vi "run_weather.vi"() -> ()   [LabVIEW 2011]
uses:
  <vilib>/xml/Load XML File.vi
  <vilib>/xml/Close Reference(Node).vi
  <vilib>/xml/NI_XML.lvlib
panel:
  out "Error Msg":string
  out "Updating Weather":bool
  out "?":picture
  out "Hourly Forecast":string[][](array[string])
  in  "Update Interval (hour)":dbl=1.0
  out "Current Weather":string[][](array[string])
  out "Observation Time (RFC 822)":string
  out "Elevation":string
  out "Longitude":string
  out "Latitude":string
  out "Country (ISO 3166)":string
  out "Location":string
  in  "City":string="stockholm"
  in  "Country":string="sweden"
  out "URL":string
  out "Key ID":string="3b63fd7c50251341"
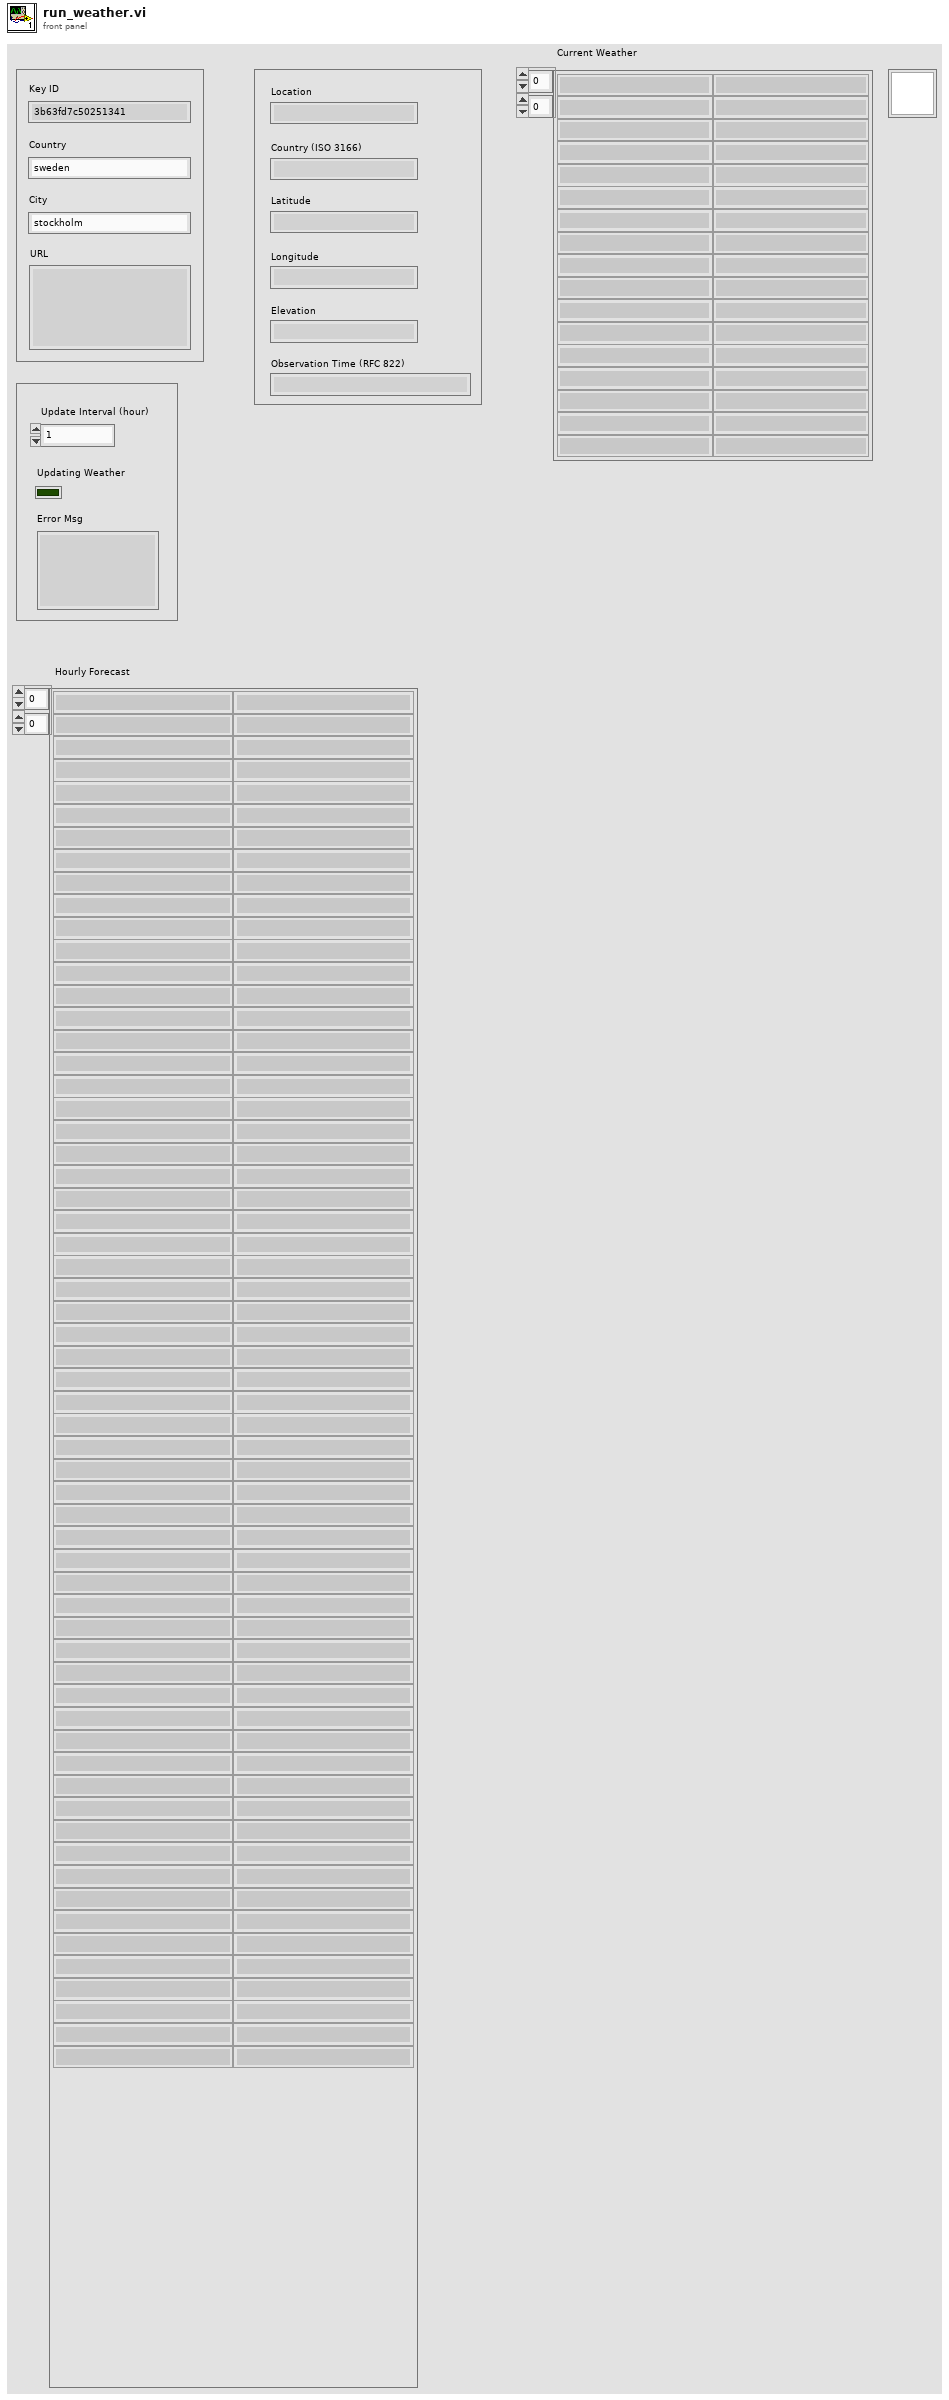
[diagram p1: front panel]
types:
  T1 = enum16{"open", "open or create", "create or replace", "create", "open (read only)"}
  T2 = typedef "imagedata.ctl" = cluster{"image type":i32, "image depth":i32, "image":u8[], "mask":u8[], "colors":u32[], "Rectangle":cluster{"left":i16, "top":i16, "right":i16, "bottom":i16}}
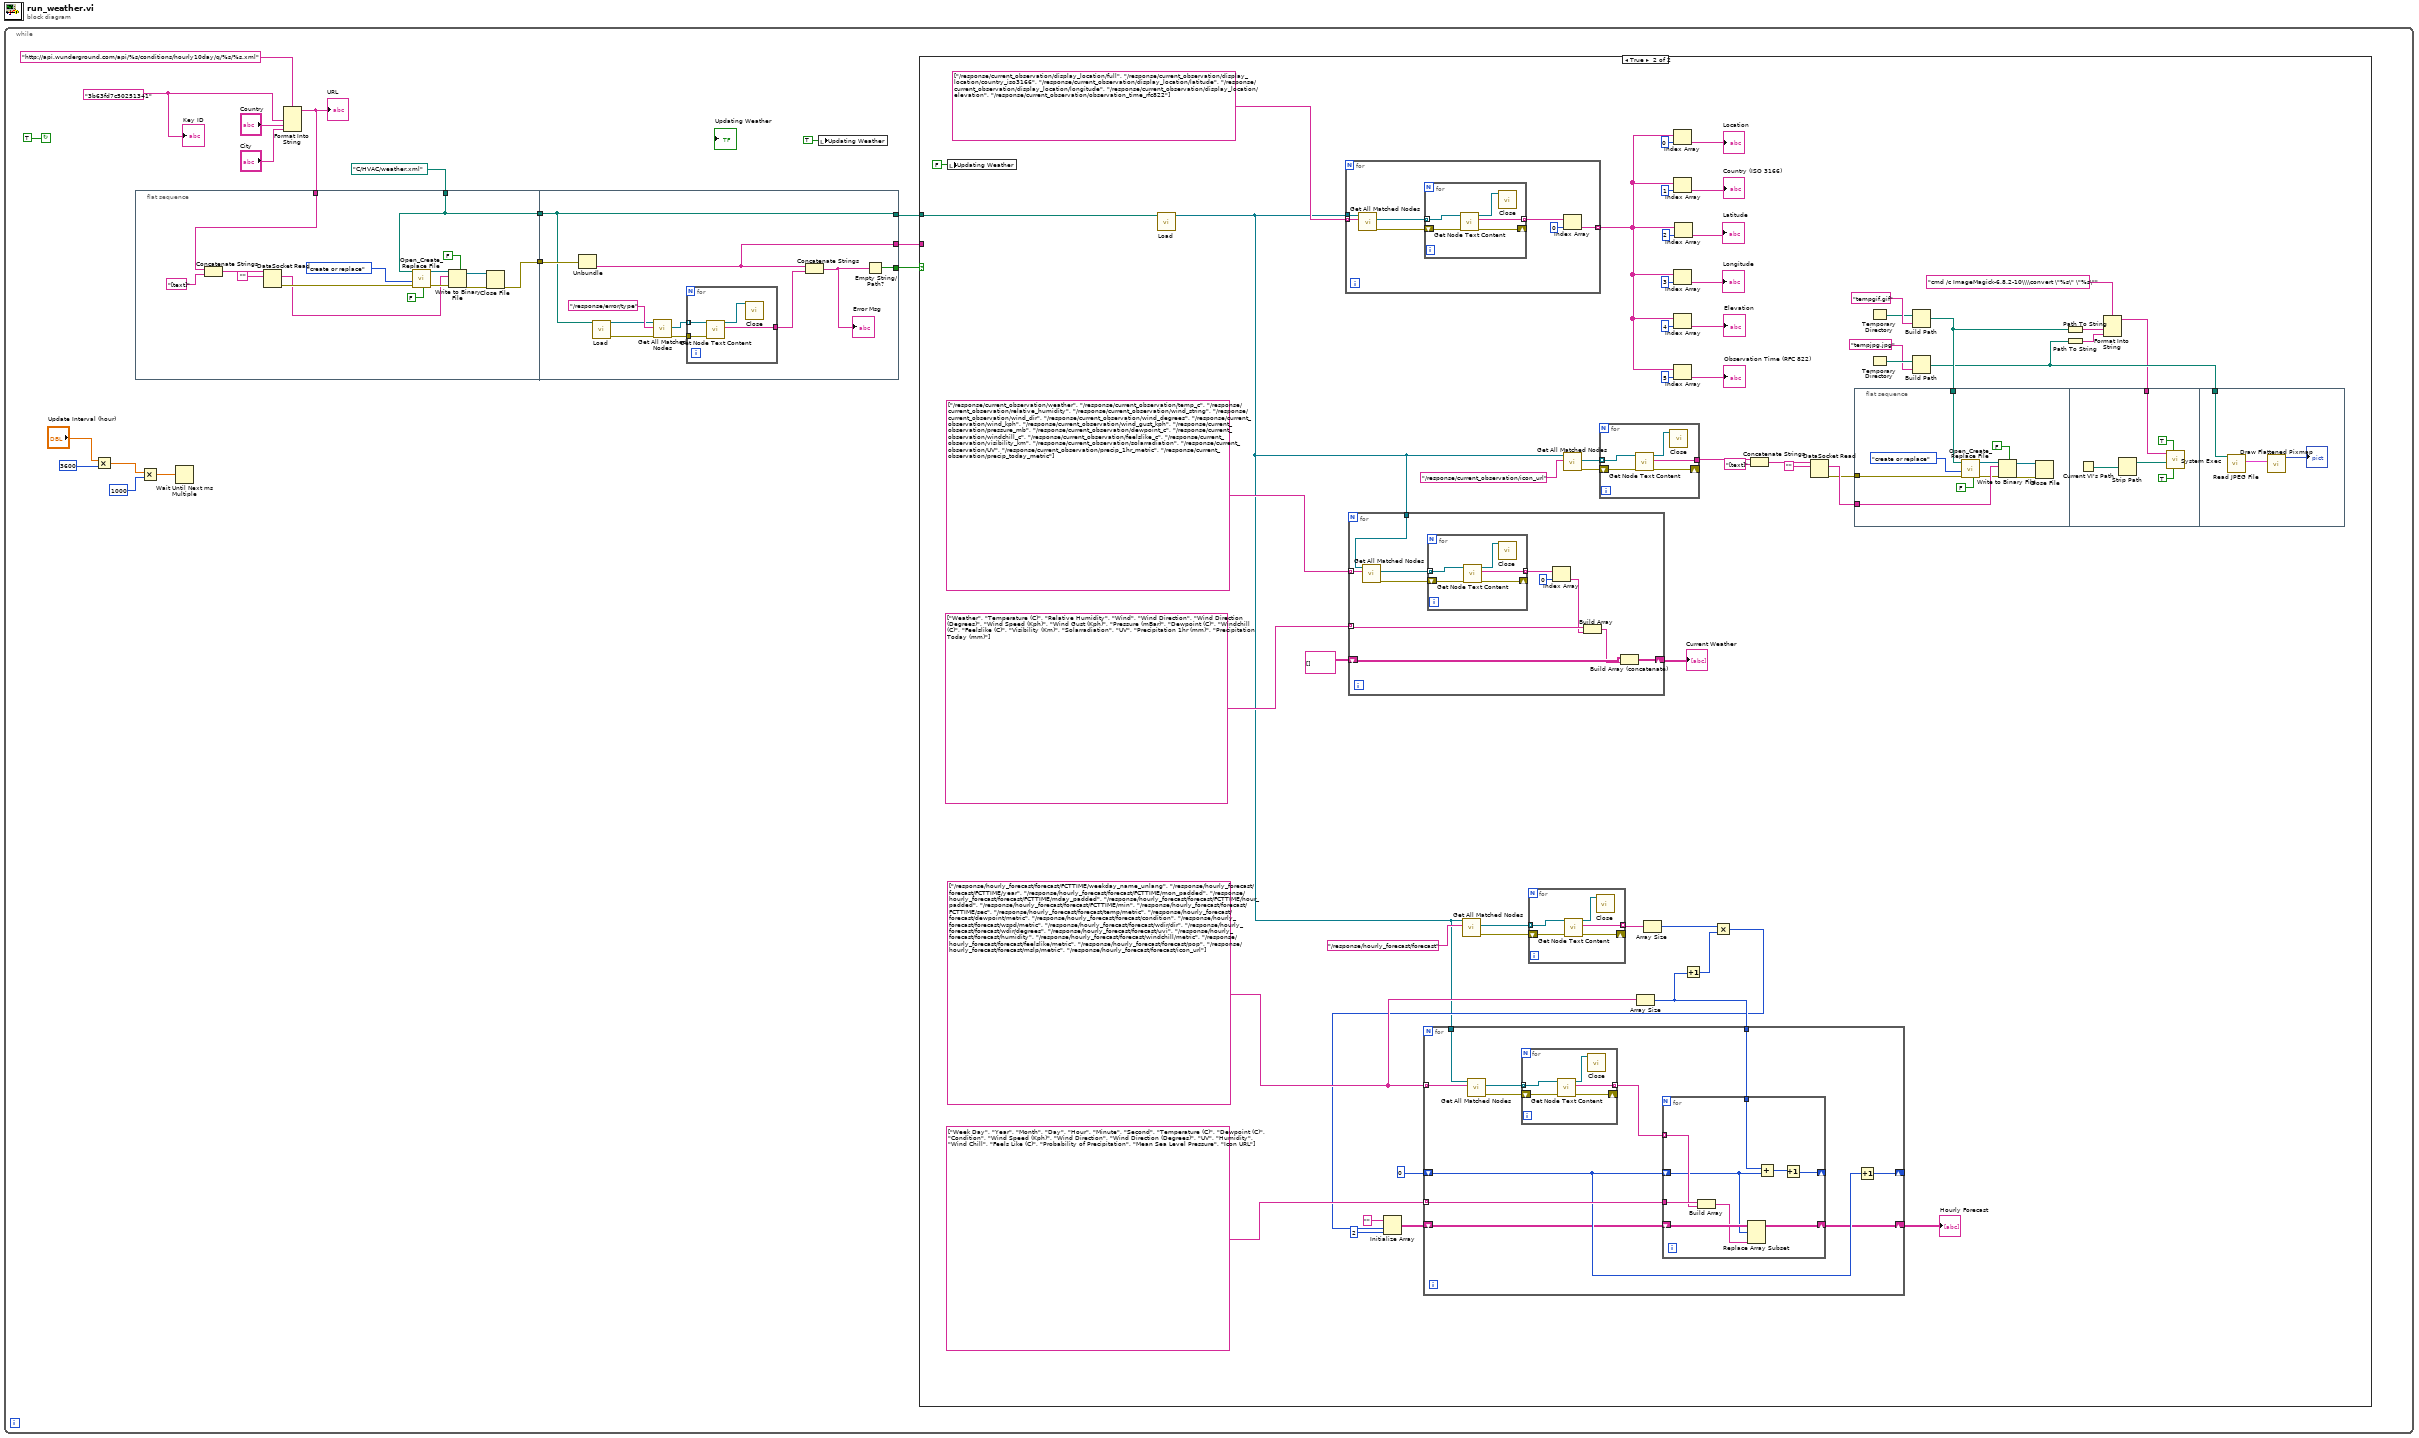
[diagram p0: block diagram]
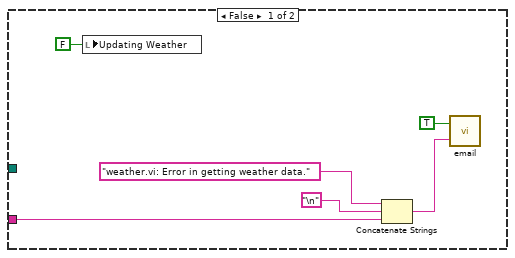
[diagram p2: hidden frame]
diagram:
  n1 = while {
    stop <- TRUE continue-if-true
    w17 = "3b63fd7c50251341"
    n2 = Multiply(x="Update Interval (hour)", y=3600) -> (x*y=w14:dbl)
    n3 = flat-sequence {
      tunnel: path "C:/HVAC/weather.xml" ("file (use dialog)") -> [w20]
      tunnel: [w20] -> w6
      tunnel: [w19] -> w5
      tunnel: w2 -> [w23]
      tunnel: w6 -> [w36]
      tunnel: w5 -> [w37]
      tunnel: [w36] -> w4
      tunnel: [w35] -> w3
      tunnel: [w34] -> w1
      frame #0 {
        n4 = Concatenate Strings(w23, "[text]" ("string")) -> (w26:string)
        n5 = DataSocket Read(10:"", 11:w26) -> (0:w22:errorcluster, 2:w21:string)  [unwired: 3 in, 5 out]
        n6 = call <vilib>:"Open_Create_Replace File.vi"("advisory dialog? (display:T)"=FALSE, "error in (no error)"=w22, "function (open:0)"=T1."create or replace", "file path"=w20) -> ("error out"=w29:errorcluster, "refnum"=w28:refnum<file>)  [unwired: 3 in, 3 out]
        n7 = Write to Binary File(file (use dialog)=w28, data=w21, error in=w29, 5:FALSE ("prepend array or string size? (T)")) -> (refnum out=w32:refnum<file>, error out=w33:errorcluster)  [unwired: 3 out]
        n8 = Close File(refnum=w32, error in=w33) -> (error out=w19:errorcluster)  [unwired: 1 out]
      }
      frame #1 {
        n9 = Unbundle(w37) -> ("source"=w34:string)  [unwired: 2 out]
        n10 = call-poly <vilib>:"Load.vi"("path to XML document"=w36) -> ("DOM document out"=w42:refnum<k20>, "error out"=w41:errorcluster)  [unwired: 12 in, 1 out]
        n11 = call <vilib>:"Get All Matched Nodes.vi"("error in (no error)"=w41, "XPath expression"="/response/error/type", "node in"=w42) -> ("error out"=w44:errorcluster, "node result array"=w40:refnum<k20>[])  [unwired: 7 out]
        n12 = for {
          tunnel: w44 -> [w48]
          tunnel: [w47] -> w38
          tunnel: w40 -> [w45] mode=indexing
          n13 = call <vilib>:"Get Node Text Content.vi"("error in (no error)"=w48, "node in"=w45) -> ("node text"=w47:string, "node out"=w46:refnum<k20>)  [unwired: 7 in, 1 out]
          n14 = call-poly <vilib>:"Close.vi"("node"=w46) -> ()  [unwired: 8 in, 1 out]
        }
        n15 = Concatenate Strings(w34, w38) -> (w39:string)
        "Error Msg" <- w39
        n16 = Empty String/Path?(string/path=w39) -> (empty?=w35:bool)
      }
    }
    n17 = Multiply(x=w14, y=1000) -> (x*y=w12:dbl)
    n18 = Wait Until Next ms Multiple(millisecond multiple=w12) -> ()  [unwired: 1 out]
    n19 = Format Into String(format string="http://api.wunderground.com/api/%s/conditions/hourly10day/q/%s/%s.xml", w17, "Country", "City") -> (resulting string=w2:string)  [unwired: 2 in, 1 out]
    "URL" <- w2
    n20 = local write "Updating Weather"(TRUE ("Backup in Progress")) -> ()
    n21 = case shown="True" w3 {
      tunnel: w4 -> [_ w109]
      tunnel: w1 -> [w50 _]
      frame False {
        n22 = local write "Updating Weather"(FALSE ("Updating Weather")) -> ()
        n23 = Concatenate Strings("weather.vi: Error in getting weather data.", "\n", w50) -> (w49:string)
        n24 = call "email.vi"("Body"=w49, "Enable"=TRUE) -> ()  [unwired: 1 in]
      }
      frame True {
        w89 = string[] ["/response/hourly_forecast/forecast/FCTTIME/weekday_name_unlang", "/response/hourly_forecast/forecast/FCTTIME/year", "/response/hourly_forecast/forecast/FCTTIME/mon_padded", "/response/hourly_forecast/forecast/FCTTIME/mday_padded", "/response/hourly_forecast/forecast/FCTTIME/hour_padded", "/response/hourly_forecast/forecast/FCTTIME/min", "/response/hourly_forecast/forecast/FCTTIME/sec", "/response/hourly_forecast/forecast/temp/metric", "/response/hourly_forecast/forecast/dewpoint/metric", "/response/hourly_forecast/forecast/condition", "/response/hourly_forecast/forecast/wspd/metric", "/response/hourly_forecast/forecast/wdir/dir", "/response/hourly_forecast/forecast/wdir/degrees", "/response/hourly_forecast/forecast/uvi", "/response/hourly_forecast/forecast/humidity", "/response/hourly_forecast/forecast/windchill/metric", "/response/hourly_forecast/forecast/feelslike/metric", "/response/hourly_forecast/forecast/pop", "/response/hourly_forecast/forecast/mslp/metric", "/response/hourly_forecast/forecast/icon_url"]
        n25 = local write "Updating Weather"(FALSE ("Backup in Progress")) -> ()
        n26 = call-poly <vilib>:"Load.vi"("path to XML document"=w109) -> ("DOM document out"=w73:refnum<k20>)  [unwired: 12 in, 2 out]
        n27 = for {
          tunnel: string[] ["/response/current_observation/display_location/full", "/response/current_observation/display_location/country_iso3166", "/response/current_observation/display_location/latitude", "/response/current_observation/display_location/longitude", "/response/current_observation/display_location/elevation", "/response/current_observation/observation_time_rfc822"] -> [w184] mode=indexing
          tunnel: w73 -> [w183]
          tunnel: [w179] -> w100 mode=indexing
          n28 = call <vilib>:"Get All Matched Nodes.vi"("XPath expression"=w184, "node in"=w183) -> ("error out"=w182:errorcluster, "node result array"=w185:refnum<k20>[])  [unwired: 1 in, 7 out]
          n29 = for {
            tunnel: w185 -> [w190] mode=indexing
            tunnel: [w189] -> w181 mode=indexing
            shift-right: [w187] -> _
            shift-left: w182 -> [w188]
            n30 = call <vilib>:"Get Node Text Content.vi"("error in (no error)"=w188, "node in"=w190) -> ("error out"=w187:errorcluster, "node text"=w189:string, "node out"=w186:refnum<k20>)  [unwired: 7 in]
            n31 = call-poly <vilib>:"Close.vi"("node"=w186) -> ()  [unwired: 8 in, 1 out]
          }
          n32 = Index Array(array=w181, index=0) -> (element=w179:string)
        }
        n33 = for {
          tunnel: string[] ["/response/current_observation/weather", "/response/current_observation/temp_c", "/response/current_observation/relative_humidity", "/response/current_observation/wind_string", "/response/current_observation/wind_dir", "/response/current_observation/wind_degrees", "/response/current_observation/wind_kph", "/response/current_observation/wind_gust_kph", "/response/current_observation/pressure_mb", "/response/current_observation/dewpoint_c", "/response/current_observation/windchill_c", "/response/current_observation/feelslike_c", "/response/current_observation/visibility_km", "/response/current_observation/solarradiation", "/response/current_observation/UV", "/response/current_observation/precip_1hr_metric", "/response/current_observation/precip_today_metric"] -> [w172] mode=indexing
          tunnel: w73 -> [w168]
          shift-right: [w165] -> w91
          shift-left: string[][] [] -> [w164]
          tunnel: string[] ["Weather", "Temperature (C)", "Relative Humidity", "Wind", "Wind Direction", "Wind Direction (Degrees)", "Wind Speed (Kph)", "Wind Gust (Kph)", "Pressure (mBar)", "Dewpoint (C)", "Windchill (C)", "Feelslike (C)", "Visibility (Km)", "Solarradiation", "UV", "Precipitation 1hr (mm)", "Precipitation Today (mm)"] -> [w167] mode=indexing
          n34 = call <vilib>:"Get All Matched Nodes.vi"("XPath expression"=w172, "node in"=w168) -> ("error out"=w171:errorcluster, "node result array"=w173:refnum<k20>[])  [unwired: 1 in, 7 out]
          n35 = for {
            tunnel: w173 -> [w178] mode=indexing
            tunnel: [w177] -> w170 mode=indexing
            shift-right: [w175] -> _
            shift-left: w171 -> [w176]
            n36 = call <vilib>:"Get Node Text Content.vi"("error in (no error)"=w176, "node in"=w178) -> ("error out"=w175:errorcluster, "node text"=w177:string, "node out"=w174:refnum<k20>)  [unwired: 7 in]
            n37 = call-poly <vilib>:"Close.vi"("node"=w174) -> ()  [unwired: 8 in, 1 out]
          }
          n38 = Index Array(array=w170, index=0) -> (element=w166:string)
          n39 = Build Array(w167, w166) -> (w163:string[])
          n40 = Build Array (concatenate)(w164, w163) -> (w165:string[][])
        }
        "Current Weather" <- w91
        n41 = call <vilib>:"Get All Matched Nodes.vi"("XPath expression"="/response/hourly_forecast/forecast", "node in"=w73) -> ("error out"=w83:errorcluster, "node result array"=w82:refnum<k20>[])  [unwired: 1 in, 7 out]
        n42 = for {
          tunnel: w82 -> [w137] mode=indexing
          tunnel: [w136] -> w80 mode=indexing
          shift-right: [w134] -> _
          shift-left: w83 -> [w135]
          n43 = call <vilib>:"Get Node Text Content.vi"("error in (no error)"=w135, "node in"=w137) -> ("error out"=w134:errorcluster, "node text"=w136:string, "node out"=w133:refnum<k20>)  [unwired: 7 in]
          n44 = call-poly <vilib>:"Close.vi"("node"=w133) -> ()  [unwired: 8 in, 1 out]
        }
        n45 = call <vilib>:"Get All Matched Nodes.vi"("XPath expression"="/response/current_observation/icon_url", "node in"=w73) -> ("error out"=w75:errorcluster, "node result array"=w74:refnum<k20>[])  [unwired: 1 in, 7 out]
        n46 = for {
          tunnel: w74 -> [w132] mode=indexing
          tunnel: [w131] -> w68
          shift-right: [w129] -> _
          shift-left: w75 -> [w130]
          n47 = call <vilib>:"Get Node Text Content.vi"("error in (no error)"=w130, "node in"=w132) -> ("error out"=w129:errorcluster, "node text"=w131:string, "node out"=w128:refnum<k20>)  [unwired: 7 in]
          n48 = call-poly <vilib>:"Close.vi"("node"=w128) -> ()  [unwired: 8 in, 1 out]
        }
        n49 = Array Size(array=w89) -> (size(s)=w79:i32)
        n50 = Array Size(array=w80) -> (size(s)=w78:i32)
        n51 = Index Array(array=w100, index=0) -> (element=→"Location":string)
        n52 = Index Array(array=w100, index=1) -> (element=→"Country (ISO 3166)":string)
        n53 = Index Array(array=w100, index=3) -> (element=→"Longitude":string)
        n54 = Index Array(array=w100, index=4) -> (element=→"Elevation":string)
        n55 = Index Array(array=w100, index=5) -> (element=→"Observation Time (RFC 822)":string)
        n56 = Index Array(array=w100, index=2) -> (element=→"Latitude":string)
        n57 = Increment(x=w79) -> (x+1=w77:i32)
        n58 = Multiply(x=w78, y=w77) -> (x*y=w76:i32)
        n59 = Initialize Array("", w76, 2 ("dimension size")) -> (w84:string[][])
        n60 = for {
          tunnel: w89 -> [w147] mode=indexing
          tunnel: w73 -> [w145]
          shift-right: [w138] -> w87
          shift-left: w84 -> [w139]
          tunnel: string[] ["Week Day", "Year", "Month", "Day", "Hour", "Minute", "Second", "Temperature (C)", "Dewpoint (C)", "Condition", "Wind Speed (Kph)", "Wind Direction", "Wind Direction (Degrees)", "UV", "Humidity", "Wind Chill", "Feels Like (C)", "Probability of Precipitation", "Mean Sea Level Pressure", "Icon URL"] -> [w142] mode=indexing
          tunnel: w79 -> [w143]
          shift-right: [w141] -> _
          shift-left: 0 -> [w140]
          n61 = call <vilib>:"Get All Matched Nodes.vi"("XPath expression"=w147, "node in"=w145) -> ("error out"=w146:errorcluster, "node result array"=w148:refnum<k20>[])  [unwired: 1 in, 7 out]
          n62 = for {
            tunnel: w148 -> [w162] mode=indexing
            tunnel: [w161] -> w144 mode=indexing
            shift-right: [w159] -> _
            shift-left: w146 -> [w160]
            n63 = call <vilib>:"Get Node Text Content.vi"("error in (no error)"=w160, "node in"=w162) -> ("error out"=w159:errorcluster, "node text"=w161:string, "node out"=w158:refnum<k20>)  [unwired: 7 in]
            n64 = call-poly <vilib>:"Close.vi"("node"=w158) -> ()  [unwired: 8 in, 1 out]
          }
          n65 = for {
            tunnel: w144 -> [w152] mode=indexing
            shift-right: [w155] -> _
            shift-left: w140 -> [w150]
            tunnel: w143 -> [w157]
            tunnel: w142 -> [w153]
            shift-right: [w149] -> w138
            shift-left: w139 -> [w154]
            n66 = Build Array(w153, w152) -> (w151:string[])
            n67 = Replace Array Subset(array=w154, new element=w151, index (row)=w150) -> (w149:string[][])  [unwired: 1 in]
            n68 = Add(x=w157, y=w150) -> (x+y=w156:i32)
            n69 = Increment(x=w156) -> (x+1=w155:i32)
          }
          n70 = Increment(x=w140) -> (x+1=w141:i32)
        }
        "Hourly Forecast" <- w87
        n71 = Concatenate Strings(w68, "[text]" ("string")) -> (w66:string)
        n72 = DataSocket Read(10:"", 11:w66) -> (0:w69:errorcluster, 2:w71:string)  [unwired: 3 in, 5 out]
        n73 = flat-sequence {
          tunnel: w71 -> [w117]
          tunnel: w69 -> [w114]
          tunnel: w61 -> [w110]
          tunnel: w56 -> [w120]
          tunnel: w58 -> [w125]
          frame #0 {
            n74 = call <vilib>:"Open_Create_Replace File.vi"("advisory dialog? (display:T)"=FALSE, "error in (no error)"=w114, "function (open:0)"=T1."create or replace", "file path"=w110) -> ("error out"=w116:errorcluster, "refnum"=w118:refnum<file>)  [unwired: 3 in, 3 out]
            n75 = Write to Binary File(file (use dialog)=w118, data=w117, error in=w116, 5:FALSE ("prepend array or string size? (T)")) -> (refnum out=w112:refnum<file>, error out=w111:errorcluster)  [unwired: 3 out]
            n76 = Close File(refnum=w112, error in=w111) -> ()  [unwired: 2 out]
          }
          frame #1 {
            n77 = Current VI's Path() -> (path=w121:path)
            n78 = Strip Path(path=w121) -> (stripped path=w124:path)  [unwired: 1 out]
            n79 = call <vilib>:"System Exec.vi"("run minimized? (F)"=TRUE, "wait until completion? (T)"=TRUE, "working directory"=w124, "command line"=w120) -> ()  [unwired: 4 in, 4 out]
          }
          frame #2 {
            n80 = call <vilib>:"Read JPEG File.vi"("path to JPEG file"=w125) -> ("image data"=w126:T2)  [unwired: 8 in, 2 out]
            n81 = call <vilib>:"Draw Flattened Pixmap.vi"("image data"=w126) -> ("new picture"=→"?":picture)  [unwired: 3 in, 5 out]
          }
        }
        n82 = Temporary Directory() -> (w64:path)
        n83 = Temporary Directory() -> (w63:path)
        n84 = Build Path(base path=w64, name or relative path="tempgif.gif") -> (appended path=w61:path)
        n85 = Build Path(base path=w63, name or relative path="tempjpg.jpg") -> (appended path=w58:path)
        n86 = Path To String(path=w61) -> (string=w60:string)
        n87 = Path To String(path=w58) -> (string=w59:string)
        n88 = Format Into String(format string="cmd /c ImageMagick-6.8.2-10\\\\convert \"%s\" \"%s\"", w60, w59) -> (resulting string=w56:string)  [unwired: 2 in, 1 out]
      }
    }
    "Key ID" <- w17
  }
